vi "balance quotes.vi"(10 "offset":i32, 11 "string":string) -> (2 "offset out":i32, 3 "quoted string":string)   [LabVIEW 2020, in "Multi Error Cluster.lvlib"]
uses:
  <vilib>/MultiError/TokenizeJSON/Multi Error Cluster.lvlib
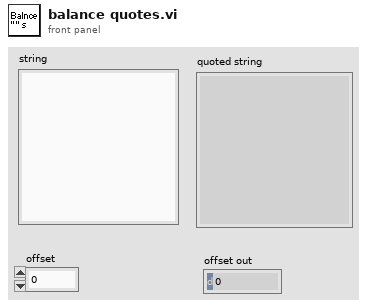
[diagram p1: front panel]
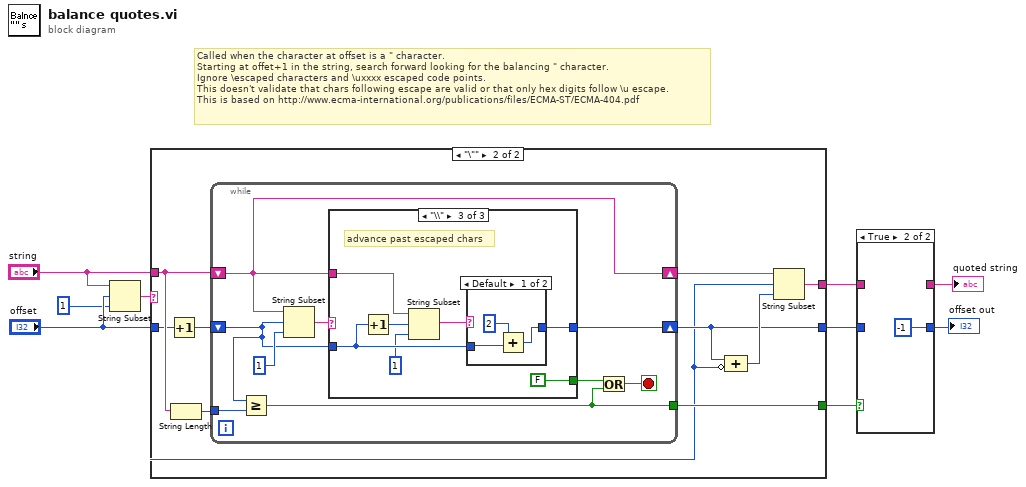
[diagram p0: block diagram]
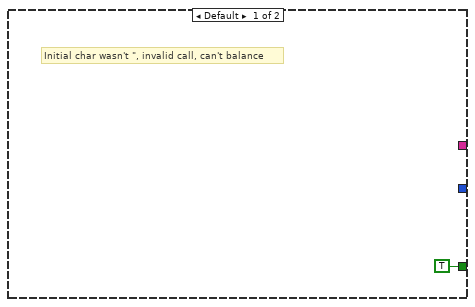
[diagram p2: hidden frame]
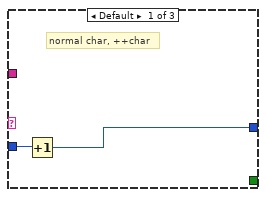
[diagram p3: hidden frame]
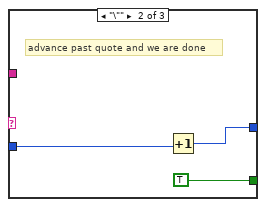
[diagram p4: hidden frame]
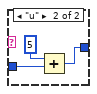
[diagram p5: hidden frame]
diagram:
  # "Called when the character at offset is a \" character.\nStarting at offet+1 in the string, search forward looking for the balancing \" character.\nIgnore \\escaped characters and \\uxxxx escaped code points.\nThis doesn't validate that chars following escape are valid or that only hex digits follow \\u escape.\nThis is based on http://www.ecma-international.org/publications/files/ECMA-ST/ECMA-404.pdf"
  n1 = String Subset(string="string", offset (0)="offset", length (rest)=1) -> (substring=w1:string)
  n2 = case shown="\"\\\"\"" w1 {
    tunnel: [_ w15] -> w9
    tunnel: [TRUE w14] -> w8
    tunnel: [_ w13] -> w5
    tunnel: "string" -> [_ w12]
    tunnel: "offset" -> [_ w11]
    frame Default {
      # "Initial char wasn't \", invalid call, can't balance"
    }
    frame "\"" {
      n3 = Increment(x=w11) -> (x+1=w19:i32)
      n4 = String Length(string=w12) -> (length=w16:i32)
      n5 = while {
        shift-right: [w24] -> w18
        shift-left: w12 -> [w24]
        shift-right: [w25] -> w13
        shift-left: w19 -> [w23]
        tunnel: w16 -> [w22]
        tunnel: [w20] -> w14
        stop <- w21 stop-if-true
        n6 = Greater Or Equal?(x=w23, y=w22) -> (x >= y?=w20:bool)
        n7 = String Subset(string=w24, offset (0)=w23, length (rest)=1) -> (substring=w27:string)
        n8 = case shown="\"\\\\\"" w27 {
          tunnel: w23 -> [w30 w32 w37]
          tunnel: [_ TRUE FALSE] -> w26
          tunnel: [w29 w31 w39] -> w25
          tunnel: w24 -> [_ _ w38]
          frame Default {
            # "normal char, ++char"
            n9 = Increment(x=w30) -> (x+1=w29:i32)
          }
          frame "\"" {
            # "advance past quote and we are done"
            n10 = Increment(x=w32) -> (x+1=w31:i32)
          }
          frame "\\" {
            # "advance past escaped chars"
            n11 = Increment(x=w37) -> (x+1=w36:i32)
            n12 = String Subset(string=w38, offset (0)=w36, length (rest)=1) -> (substring=w34:string)
            n13 = case shown="Default" w34 {
              tunnel: w37 -> [w42 w46]
              tunnel: [w41 w45] -> w39
              frame Default {
                n14 = Add(x=2, y=w42) -> (x+y=w41:i32)
              }
              frame "u" {
                n15 = Add(x=5, y=w46) -> (x+y=w45:i32)
              }
            }
          }
        }
        n16 = Or(x=w26, y=w20) -> (x .or. y?=w21:bool)
      }
      n17 = Compound Arithmetic op=ADD(w13, invert w11) -> (w17:i32)
      n18 = String Subset(string=w18, offset (0)=w11, length (rest)=w17) -> (substring=w15:string)
    }
  }
  n19 = case shown="True" w8 {
    tunnel: w9 -> [w48 _]
    tunnel: [w48 _] -> w7
    tunnel: [w47 -1] -> w6
    tunnel: w5 -> [w47 _]
    frame False {
    }
    frame True {
    }
  }
  "offset out" <- w6
  "quoted string" <- w7
